vi "sub_num-to-color.vi"(11 "ratio":dbl) -> (3 "color num":u32)   [LabVIEW 2019]
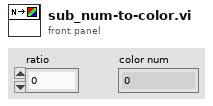
[diagram p1: front panel]
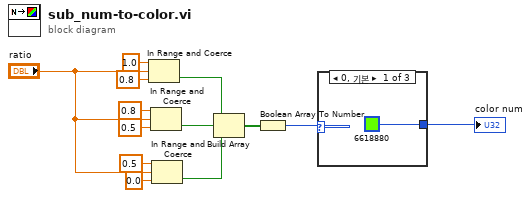
[diagram p0: block diagram]
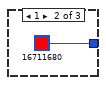
[diagram p2: hidden frame]
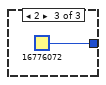
[diagram p3: hidden frame]
diagram:
  n1 = In Range and Coerce(upper limit=1.0, x="ratio", lower limit=0.8) -> (In Range?=w3:bool)  [unwired: 1 out]
  n2 = In Range and Coerce(upper limit=0.8, x="ratio", lower limit=0.5) -> (In Range?=w12:bool)  [unwired: 1 out]
  n3 = In Range and Coerce(upper limit=0.5, x="ratio", lower limit=0.0) -> (In Range?=w11:bool)  [unwired: 1 out]
  n4 = Build Array(w3, w12, w11) -> (w13:bool[])
  n5 = Boolean Array To Number(Boolean array=w13) -> (number=w2:u32)
  n6 = case shown="0, 기본" w2 {
    tunnel: [u32 6618880 ("blue") u32 16711680 ("red") u32 16776072 ("Y")] -> w1
    frame 0, Default {
    }
    frame 1 {
    }
    frame 2 {
    }
  }
  "color num" <- w1
